vi "VDH-init.vi"(8 "error in (no error)":errorcluster, 11 "VDH-VNA_data_handler in":refnum<class "VDH-VNA_data_handler.lvclass">) -> (0 "error out":errorcluster, 3 "VDH-VNA_data_handler out":refnum<class "VDH-VNA_data_handler.lvclass">)   [LabVIEW 2020, in "VDH-VNA_data_handler.lvlib" / "VDH-VNA_data_handler.lvclass"]
uses:
  VDH-VNA_data_handler.lvclass
  C:/Program Files (x86)/National Instruments/LabVIEW 2020/vi.lib/ActorFramework/Actor/Actor.lvclass
  <vilib>/ActorFramework/Actor/Actor.lvclass/Actor.ctl
  <vilib>/ActorFramework/Message Enqueuer/Message Enqueuer.lvclass/Message Enqueuer.ctl
  VDH-VNA_data_handler.lvclass/VDH-VNA_data_handler.ctl
  hardware_manager/VHM-VNA_Hardware_Manager/VHM-VNA_Hardware_Manager Messages/VHM-transferVDHEnqueue Msg/VHM-transferVDHEnqueue Msg.lvclass/VHM-transferVDHEnqueue Msg.ctl
  VDHI-VNA_data_handler_interface Messages/VHDI-recieveCalibrationStatus Msg/VHDI-recieveCalibrationStatus Msg.lvclass/VHDI-recieveCalibrationStatus Msg.ctl
  <vilib>/ActorFramework/Message Enqueuer/Init from Existing Queue.vi
  <vilib>/ActorFramework/Message Enqueuer/Enqueue.vi
  hardware_manager/VHM-VNA_Hardware_Manager/VHM-VNA_Hardware_Manager Messages/VHM-transferVDHEnqueue Msg/VHM-transferVDHEnqueue Msg.lvclass
  C:/Program Files (x86)/National Instruments/LabVIEW 2020/vi.lib/ActorFramework/Message/Message.lvclass
  VDHI-VNA_data_handler_interface Messages/VHDI-recieveCalibrationStatus Msg/VHDI-recieveCalibrationStatus Msg.lvclass
  <vilib>/ActorFramework/Message Priority Queue/Priority Enqueue.vi
  <vilib>/ActorFramework/Message Enqueuer/Message Enqueuer.lvclass
  <vilib>/ActorFramework/Actor/Actor.lvclass
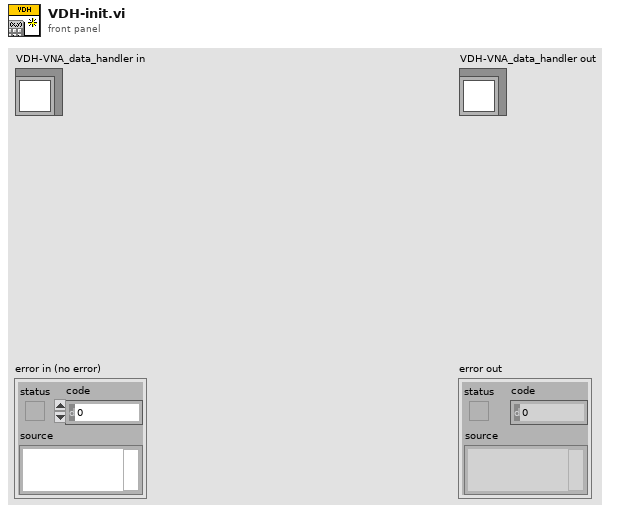
[diagram p1: front panel]
types:
  T1 = typedef "VDH-VNA_data_handler.lvlib/VDH-VNA_data_handler.lvclass/VDH-calibration_status.ctl" = cluster{"Calib Status":T2, "Calibrated?":bool, "Permativity?":bool, "Progress":T3}
  T2 = typedef "VDH-VNA_data_handler.lvlib/VDH-VNA_data_handler.lvclass/VDH-SOLT_calib_Status.ctl" = cluster{"Short":bool, "Open":bool, "Load":bool, "Through":bool}
  T3 = typedef "VDH-VNA_data_handler.lvlib/VDH-VNA_data_handler.lvclass/VDH-Calibration_prosess.ctl" = cluster{"Progress":bool, "current":T4, "samples to get":u8}
  T4 = typedef "VDH-VNA_data_handler.lvlib/VDH-VNA_data_handler.lvclass/VDH-Calibration_enum.ctl" = enum16{"Non", "Short", "Open", "Load", "Through", "Permativity"}
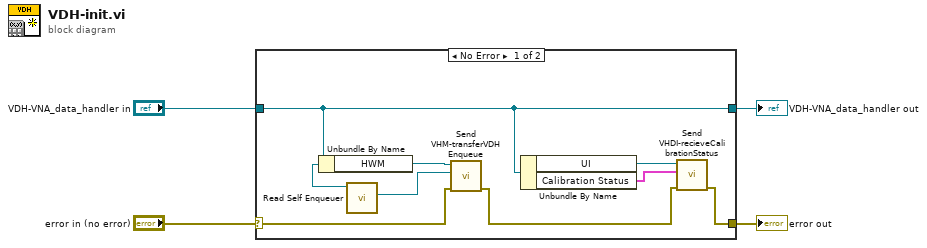
[diagram p0: block diagram]
diagram:
  n1 = case shown="No Error" "error in (no error)" {
    selector: "error in (no error)" -> [w10 w14]
    tunnel: [w5 w14] -> w3
    tunnel: [w9 w13] -> w1
    tunnel: "VDH-VNA_data_handler in" -> [w9 w13]
    frame No Error {
      n2 = Unbundle By Name(w9) -> ("HWM"=w12:refnum<class "Message Enqueuer.lvclass">)
      n3 = call <vilib>:"Read Self Enqueuer.vi"("Actor"=w9) -> ("Self Enqueuer"=w11:refnum<class "Message Enqueuer.lvclass">)  [unwired: 10 in]
      n4 = call "Send VHM-transferVDHEnqueue.vi"("error in (no error)"=w10, "VDH"=w11, "Message Enqueuer"=w12) -> ("error out"=w6:errorcluster)  [unwired: 7 in, 1 out]
      n5 = Unbundle By Name(w9) -> ("UI"=w8:refnum<class "Message Enqueuer.lvclass">, "Calibration Status"=w7:T1)
      n6 = call "Send VHDI-recieveCalibrationStatus.vi"("error in (no error)"=w6, "Calibration Status"=w7, "Message Enqueuer"=w8) -> ("error out"=w5:errorcluster)  [unwired: 7 in, 1 out]
    }
    frame Error {
    }
  }
  "error out" <- w3
  "VDH-VNA_data_handler out" <- w1
